vi "_attribute_read_boolean.vi"(5 "Repeated Capability":string, 7 "Attribute":T1={"Identifier"="", "Descriptive Name"="", "Data Type"=enum."Integer 32", "Command"="", "Access"=enum."Read/Write", "Range Table"="", "Read Callback"="", "Write Callback"="", "Supported Models"="", "Instrument Options"="", "Index"=0, "OPC Wait"=FALSE, "No Status Check"=FALSE, "Cache Only"=FALSE}, 8 "error in":errorcluster caption="error in (no error)", 10 "Query Parameter":string, 11 "VISA resource name":refnum<visa-resource-name>) -> (0 "error out":errorcluster, 2 "Boolean out":bool, 3 "VISA resource name out":refnum<visa-resource-name>)   [LabVIEW 2020, in "Rohde&Schwarz RTx Oscilloscopes.lvlib" / "rsidr_core.lvlib"]
uses:
  rsidr_core.lvlib
  type_Attribute.ctl
  type_Attribute_Data_Type.ctl
  type_ReadWriteAccess.ctl
  Rohde&Schwarz RTx Oscilloscopes.lvlib
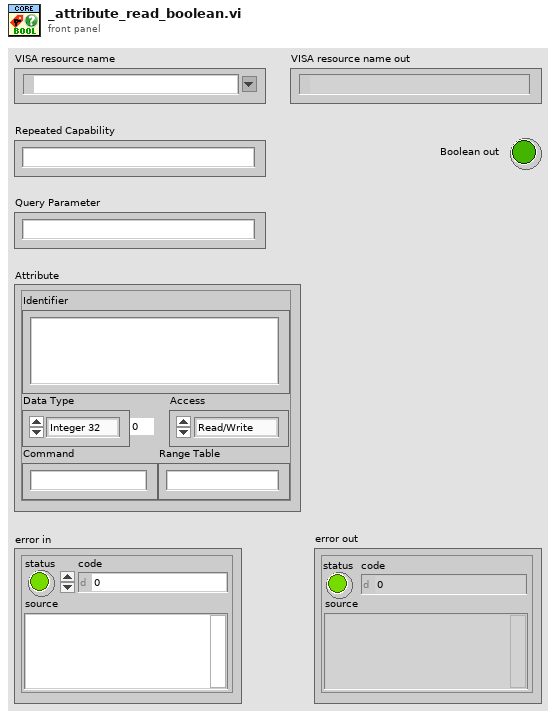
[diagram p1: front panel]
types:
  T1 = typedef "Rohde&Schwarz RTx Oscilloscopes.lvlib/rsidr_core.lvlib/type_Attribute.ctl" = cluster{"Identifier":string, "Descriptive Name":string, "Data Type":T2, "Command":string, "Access":T3, "Range Table":string, "Read Callback":string, "Write Callback":string, "Supported Models":string, "Instrument Options":string, "Index":i32, "OPC Wait":bool, "No Status Check":bool, "Cache Only":bool}
  T2 = typedef "Rohde&Schwarz RTx Oscilloscopes.lvlib/rsidr_core.lvlib/type_Attribute_Data_Type.ctl" = enum16{"Integer 32", "Double", "String", "Boolean", "None", "Integer 64", "RawString"}
  T3 = typedef "Rohde&Schwarz RTx Oscilloscopes.lvlib/rsidr_core.lvlib/type_ReadWriteAccess.ctl" = enum16{"Read Only", "Write Only", "Read/Write"}
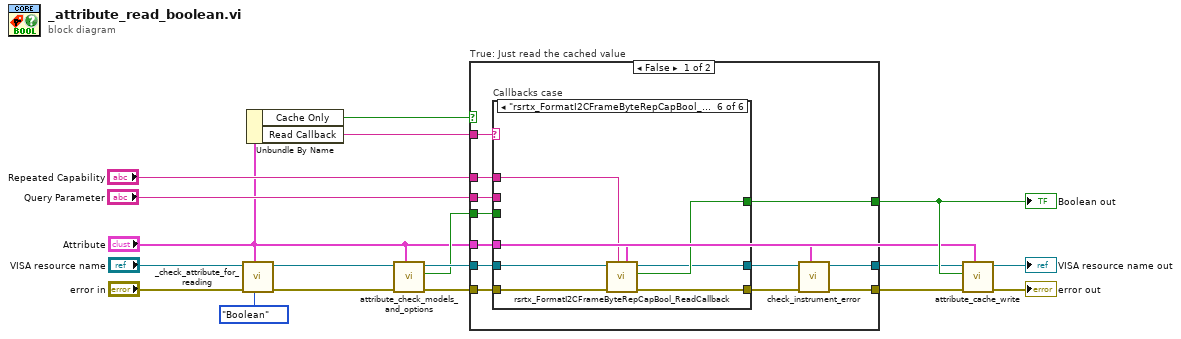
[diagram p0: block diagram]
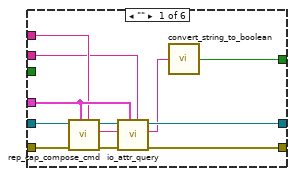
[diagram p2: hidden frame]
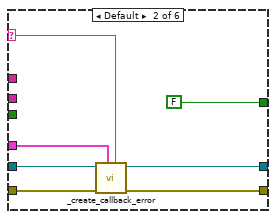
[diagram p3: hidden frame]
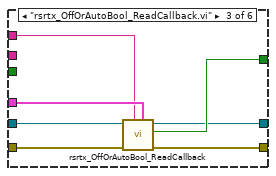
[diagram p4: hidden frame]
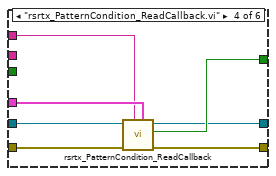
[diagram p5: hidden frame]
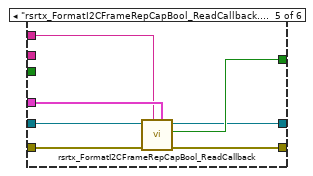
[diagram p6: hidden frame]
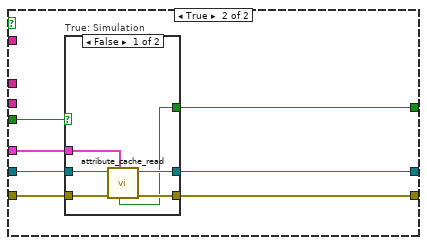
[diagram p7: hidden frame]
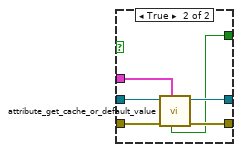
[diagram p8: hidden frame]
diagram:
  n1 = call "_check_attribute_for_reading.vi"("Expected Data Type"=type_Attribute_Data_Type."Boolean" ("Data Type"), "Attribute"="Attribute", "error in"="error in", "VISA resource name"="VISA resource name") -> ("error out"=w9:errorcluster, "VISA resource name out"=w8:refnum<visa-resource-name>)  [unwired: 6 in]
  n2 = Unbundle By Name("Attribute") -> ("Cache Only"=w1:bool, "Read Callback"=w10:string)
  n3 = call "attribute_check_models_and_options.vi"("Attribute"="Attribute", "error in"=w9, "VISA resource name"=w8) -> ("error out"=w7:errorcluster, "Simulation Mode"=w5:bool, "VISA resource name out"=w6:refnum<visa-resource-name>)  [unwired: 6 in]
  n4 = case "True: Just read the cached value" shown="False" w1 {
    tunnel: "Repeated Capability" -> [w30 _]
    tunnel: [w21 w81] -> w4
    tunnel: [w29 w78] -> w15
    tunnel: w10 -> [w28 _]
    tunnel: w6 -> [w27 w84]
    tunnel: w7 -> [w26 w83]
    tunnel: "Attribute" -> [w19 w79]
    tunnel: w5 -> [w25 w80]
    tunnel: [w20 w82] -> w3
    tunnel: "Query Parameter" -> [w24 _]
    frame False {
      n5 = case "Callbacks case" shown="\"rsrtx_FormatI2CFrameByteRepCapBool_ReadCallback.vi\"" w28 {
        selector: w28 -> [_ w44 _ _ _ _]
        tunnel: w27 -> [w42 w48 w55 w62 w69 w76]
        tunnel: w26 -> [w41 w49 w56 w63 w70 w77]
        tunnel: w30 -> [w35 _ w53 w60 w67 w74]
        tunnel: [w40 w46 w50 w57 w64 w71] -> w22
        tunnel: [w34 w47 w51 w58 w65 w72] -> w23
        tunnel: [w33 FALSE ("Attribute Value Boolean") w52 w59 w66 w73] -> w29
        tunnel: w19 -> [w36 w45 w54 w61 w68 w75]
        tunnel: w25 -> [_ _ _ _ _ _]
        tunnel: w24 -> [w31 _ _ _ _ _]
        frame "" {
          n6 = call "rep_cap_compose_cmd.vi"("Repeated Capability"=w35, "Attribute"=w36, "error in"=w41, "VISA resource name"=w42) -> ("error out"=w39:errorcluster, "Command out"=w38:string, "VISA resource name out"=w37:refnum<visa-resource-name>)  [unwired: 5 in]
          n7 = call "io_attr_query.vi"("Query Parameter (None)"=w31, "Attribute"=w36, "error in"=w39, "write buffer"=w38, "VISA resource name"=w37) -> ("error out"=w34:errorcluster, "read buffer"=w32:string, "VISA resource name out"=w40:refnum<visa-resource-name>)  [unwired: 4 in]
          n8 = call "convert_string_to_boolean.vi"("String in"=w32) -> ("boolean value out"=w33:bool)  [unwired: 4 in]
        }
        frame Default {
          n9 = call "_create_callback_error.vi"("Callback Name"=w44, "Attribute"=w45, "error in"=w49, "VISA resource name"=w48) -> ("error out"=w47:errorcluster, "VISA resource name out"=w46:refnum<visa-resource-name>)  [unwired: 6 in]
        }
        frame "rsrtx_OffOrAutoBool_ReadCallback.vi" {
          n10 = call "rsrtx_OffOrAutoBool_ReadCallback.vi"("Attribute"=w54, "Repeated Capability"=w53, "error in"=w56, "VISA resource name"=w55) -> ("error out"=w51:errorcluster, "Attribute Value Boolean"=w52:bool, "VISA resource name out"=w50:refnum<visa-resource-name>)  [unwired: 5 in]
        }
        frame "rsrtx_PatternCondition_ReadCallback.vi" {
          n11 = call "rsrtx_PatternCondition_ReadCallback.vi"("Attribute"=w61, "Repeated Capability"=w60, "error in"=w63, "VISA resource name"=w62) -> ("error out"=w58:errorcluster, "Attribute Value Boolean"=w59:bool, "VISA resource name out"=w57:refnum<visa-resource-name>)  [unwired: 5 in]
        }
        frame "rsrtx_FormatI2CFrameRepCapBool_ReadCallback.vi" {
          n12 = call "rsrtx_FormatI2CFrameRepCapBool_ReadCallback.vi"("Attribute"=w68, "Repeated Capability"=w67, "error in"=w70, "VISA resource name"=w69) -> ("error out"=w65:errorcluster, "Attribute Value Boolean"=w66:bool, "VISA resource name out"=w64:refnum<visa-resource-name>)  [unwired: 5 in]
        }
        frame "rsrtx_FormatI2CFrameByteRepCapBool_ReadCallback.vi" {
          n13 = call "rsrtx_FormatI2CFrameByteRepCapBool_ReadCallback.vi"("Attribute"=w75, "Repeated Capability"=w74, "error in"=w77, "VISA resource name"=w76) -> ("error out"=w72:errorcluster, "Attribute Value Boolean"=w73:bool, "VISA resource name out"=w71:refnum<visa-resource-name>)  [unwired: 5 in]
        }
      }
      n14 = call "check_instrument_error.vi"("Attribute"=w19, "error in"=w23, "VISA resource name"=w22) -> ("error out"=w21:errorcluster, "VISA resource name out"=w20:refnum<visa-resource-name>)  [unwired: 7 in]
    }
    frame True {
      n15 = case "True: Simulation" shown="False" w80 {
        tunnel: w83 -> [w90 w96]
        tunnel: w84 -> [w89 w95]
        tunnel: w79 -> [w88 w92]
        tunnel: [w87 w94] -> w81
        tunnel: [w86 w93] -> w82
        tunnel: [w85 w91] -> w78
        frame False {
          n16 = call "attribute_cache_read.vi"("Attribute"=w88, "error in"=w90, "VISA resource name"=w89) -> ("error out"=w87:errorcluster, "VISA resource name out"=w86:refnum<visa-resource-name>, "Boolean out"=w85:bool)  [unwired: 1 in, 5 out]
        }
        frame True {
          n17 = call "attribute_get_cache_or_default_value.vi"("Attribute"=w92, "error in"=w96, "VISA resource name"=w95) -> ("error out"=w94:errorcluster, "VISA resource name out"=w93:refnum<visa-resource-name>, "Boolean out"=w91:bool)  [unwired: 1 in, 5 out]
        }
      }
    }
  }
  "Boolean out" <- w15
  n18 = call "attribute_cache_write.vi"("Attribute"="Attribute", "error in"=w4, "Value in"=w15, "VISA resource name"=w3) -> ("error out"=→"error out":errorcluster, "VISA resource name out"=→"VISA resource name out":refnum<visa-resource-name>)  [unwired: 6 in]
